vi "CAN payload to string.vi"() -> ()   [LabVIEW 2023, in "Decoder.lvlib"]
uses:
  Project-Based-Learning/Decoder/Decoder.lvlib
panel:
  out "error out":errorcluster
  in  "error in (no error)":errorcluster
  in  "payload":u8[](array[numeric])=[3, 0, 7, 0, 255]
  out "Payload String":string
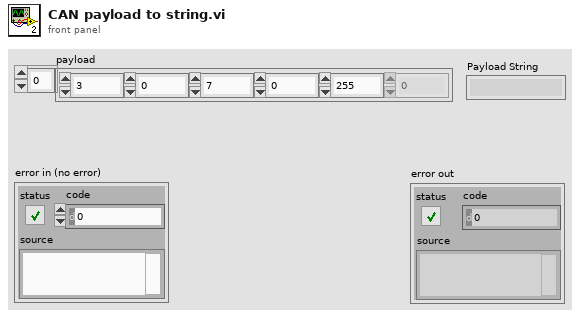
[diagram p1: front panel]
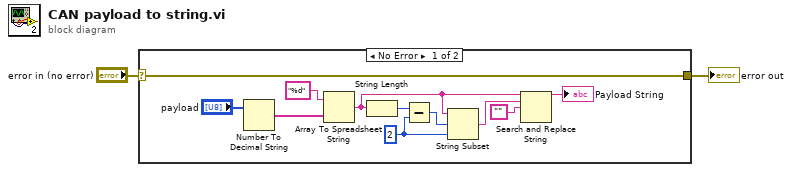
[diagram p0: block diagram]
diagram:
  n1 = case shown="No Error" "error in (no error)" {
    selector: "error in (no error)" -> [w3 w14]
    tunnel: [w3 w14] -> w1
    frame No Error {
      w9 = 2 ("y")
      n2 = Number To Decimal String(number="payload") -> (decimal integer string=w12:string[])  [unwired: 1 in]
      n3 = Array To Spreadsheet String(array=w12, 3:"%d" ("format string")) -> (spreadsheet string=w7:string)  [unwired: 1 in]
      n4 = String Length(string=w7) -> (length=w10:i32)
      n5 = Subtract(x=w10, y=w9) -> (x-y=w8:i32)
      n6 = String Subset(string=w7, offset (0)=w8, length (rest)=w9) -> (substring=w4:string)
      n7 = Search and Replace String(input string=w7, search string=w4, replace string="") -> (result string=→"Payload String":string)  [unwired: 5 in, 3 out]
    }
    frame Error {
    }
  }
  "error out" <- w1
